vi "Download with Progress and Abort.vi"() -> ()   [LabVIEW 2019]
uses:
  <vilib>/httpClient/LabVIEWHTTPClient.lvlib
panel:
  out "bytes downloaded":i64
  out "file size (bytes)":i64
  out "progress":dbl(slide) scale=0.0..100.0
  out "error out":errorcluster
  in  "Abort":bool
  in  "Folder to save file":path=path ""
  in  "file url":string
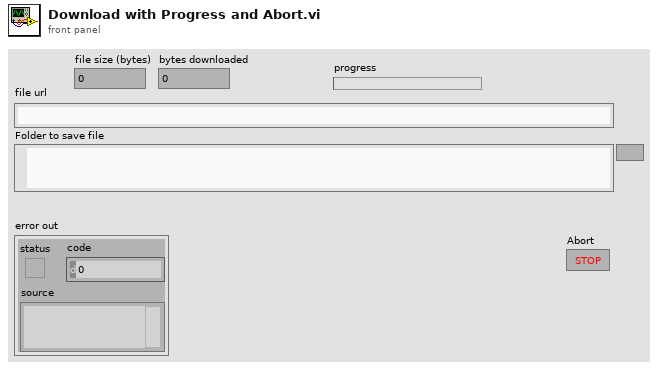
[diagram p1: front panel]
types:
  T1 = typedef "LabVIEWHTTPClient.lvlib/ClientHandle.ctl" = refnum<k1>
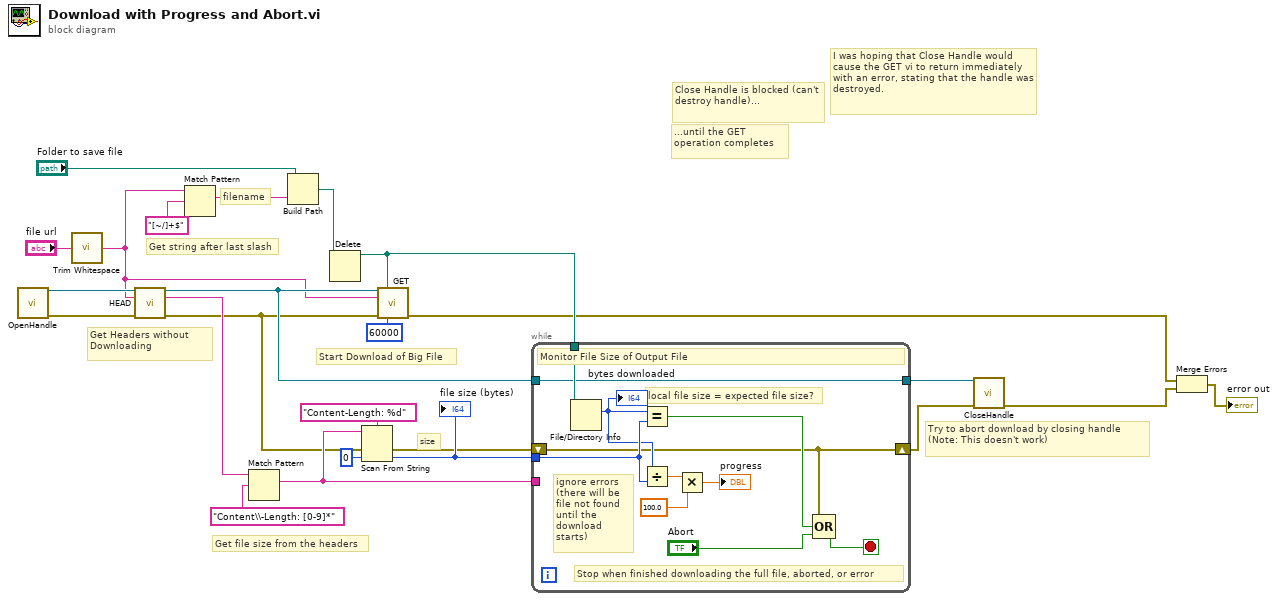
[diagram p0: block diagram]
diagram:
  # "Get string after last slash"
  # "filename"
  # "Try to abort download by closing handle\n(Note: This doesn't work)"
  # "I was hoping that Close Handle would cause the GET vi to return immediately with an error, stating that the handle was destroyed."
  # "...until the GET operation completes"
  # "Close Handle is blocked (can't destroy handle)..."
  # "size"
  # "Get file size from the headers"
  # "Start Download of Big File"
  # "Get Headers without Downloading"
  n1 = call <vilib>:"OpenHandle.vi"() -> ("client handle out"=w23:T1, "error out"=w24:errorcluster)  [unwired: 14 in]
  n2 = call <vilib>:"Trim Whitespace.vi"("string"="file url") -> ("trimmed string"=w1:string)  [unwired: 1 in]
  n3 = call <vilib>:"HEAD.vi"("client handle"=w23, "url"=w1, "error in (no error)"=w24) -> ("client handle out"=w16:T1, "headers"=w22:string, "error out"=w9:errorcluster)  [unwired: 10 in]
  n4 = Match Pattern(string=w1, regular expression="[~/]+$") -> (match substring=w4:string)  [unwired: 1 in, 3 out]
  n5 = Match Pattern(string=w22, regular expression="Content\\-Length: [0-9]*") -> (match substring=w20:string)  [unwired: 1 in, 3 out]
  n6 = Build Path(base path="Folder to save file", name or relative path=w4) -> (appended path=w2:path)
  n7 = Delete(path (use dialog)=w2) -> (deleted path=w14:path)  [unwired: 4 in, 2 out]
  n8 = Scan From String(format string="Content-Length: %d", input string=w20, error in=w9, default 1=i64 0 ("default value 1")) -> (error out=w8:errorcluster, output 1=w18:i64)  [unwired: 1 in, 2 out]
  "file size (bytes)" <- w18
  n9 = call <vilib>:"GET.vi"("client handle"=w16, "output file"=w14, "url"=w1, "error in (no error)"=w9, "timeout (10000)"=60000) -> ("error out"=w12:errorcluster)  [unwired: 7 in, 3 out]
  n10 = while {
    tunnel: w14 -> [w35]
    tunnel: w20 -> [_]
    tunnel: w18 -> [w32]
    tunnel: [w27] -> w15
    tunnel: w16 -> [w27]
    shift-right: [w25] -> w7
    shift-left: w8 -> [w25]
    stop <- w30 stop-if-true
    # "ignore errors\n(there will be file not found until the download starts)"
    # "Stop when finished downloading the full file, aborted, or error"
    # "local file size = expected file size?"
    # "Monitor File Size of Output File"
    n11 = File/Directory Info(path=w35) -> (size=w26:i64)  [unwired: 1 in, 6 out]
    "bytes downloaded" <- w26
    n12 = Equal?(x=w26, y=w32) -> (x = y?=w31:bool)
    n13 = Divide(x=w26, y=w32) -> (x/y=w34:dbl)
    n14 = Multiply(x=w34, y=100.0) -> (x*y=→"progress":dbl)
    n15 = Compound Arithmetic op=OR(w25, w31, "Abort") -> (w30:bool)
  }
  n16 = call <vilib>:"CloseHandle.vi"("client handle"=w15, "error in (no error)"=w7) -> ("error out"=w11:errorcluster)  [unwired: 13 in]
  n17 = Merge Errors(w12, w11) -> (→"error out":errorcluster)
